vi "sub_calc-2-gol-cost.vi"(8 "error in":errorcluster) -> (0 "error out":errorcluster, 3 "cost":dbl)   [LabVIEW 2019]
uses:
  Ctrl/cmd_common.ctl
panel:
  out "error angle":dbl
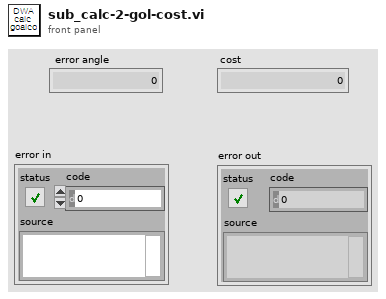
[diagram p1: front panel]
types:
  T1 = typedef "cmd_common.ctl" = enum16{"read", "write"}
  T2 = cluster{"x":dbl[], "dw":dbl[], "u":cluster{"v":dbl, "y":dbl}, "trajectory":dbl[][], "best trajectory":dbl[][], "best u":cluster{"v":dbl, "y":dbl}}
  T3 = cluster{"max speed":dbl, "min speed":dbl, "max yaw rate":dbl, "max accel":dbl, "max delta yaw rate":dbl, "v resolution":dbl, "yaw rate resolution":dbl, "dt":dbl, "predict time":dbl, "to goal cost gain":dbl, "speed cost gain":dbl, "obstacle cost gain":dbl, "robot stuck flag cons":dbl, "robot type":enum16{"circle", "rectangle"}, "robot radius":dbl, "robot width":dbl, "robot length":dbl, "obstacles":cluster{"x":dbl, "y":dbl}[], "goal pt":cluster{"x":i32, "y":i32}}
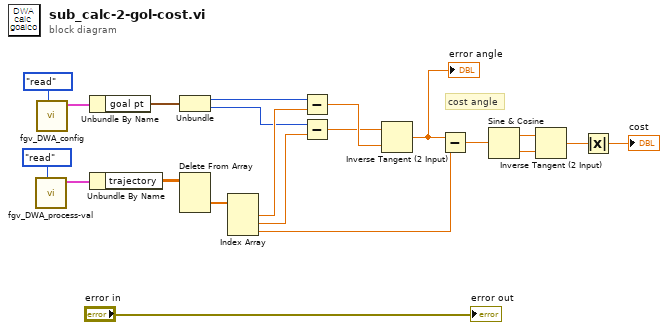
[diagram p0: block diagram]
diagram:
  # "cost angle"
  n1 = call "fgv_DWA_process-val.vi"("cmd"=cmd_common."read") -> ("prcess val out"=w20:T2)  [unwired: 10 in]
  n2 = call "fgv_DWA_config.vi"("cmd"=cmd_common."read") -> ("config out"=w18:T3)  [unwired: 10 in]
  n3 = Unbundle By Name(w18) -> ("goal pt"=w17:cluster{"x":i32, "y":i32})
  n4 = Unbundle By Name(w20) -> ("trajectory"=w16:dbl[][])
  n5 = Unbundle(w17) -> ("x"=w14:i32, "y"=w2:i32)
  n6 = Delete From Array(array=w16) -> (deleted portion=w15:dbl[])  [unwired: 3 in, 1 out]
  n7 = Index Array(array=w15) -> (element #1=w13:dbl, element #2=w3:dbl, element #3=w9:dbl)  [unwired: 3 in]
  n8 = Subtract(x=w14, y=w13) -> (x-y=w12:dbl)
  n9 = Subtract(x=w2, y=w3) -> (x-y=w11:dbl)
  n10 = Inverse Tangent (2 Input)(1:w12, 2:w11) -> (0:w10:dbl)
  "error angle" <- w10
  n11 = Subtract(x=w10, y=w9) -> (x-y=w8:dbl)
  n12 = Sine & Cosine(0:w8) -> (1:w7:dbl, 2:w6:dbl)
  n13 = Inverse Tangent (2 Input)(1:w6, 2:w7) -> (0:w5:dbl)
  n14 = Absolute Value(x=w5) -> (abs(x)=→"cost":dbl)
  "error out" <- "error in"
